vi "Get_DeviceInformation.vi"(8 "error in (no error)":errorcluster, 11 "Avantes in":refnum<class "Avantes.lvclass">) -> (0 "error out":errorcluster, 2 "Array":string[](array[string]), 3 "Avantes out":refnum<class "Avantes.lvclass">)   [LabVIEW 2020, in "Avantes.lvclass"]
uses:
  <instrlib>/Classes/CCD/Avantes/Avantes.lvclass
panel:
  in  "Enum":enum16{"Intern", "Extern"}(ring)
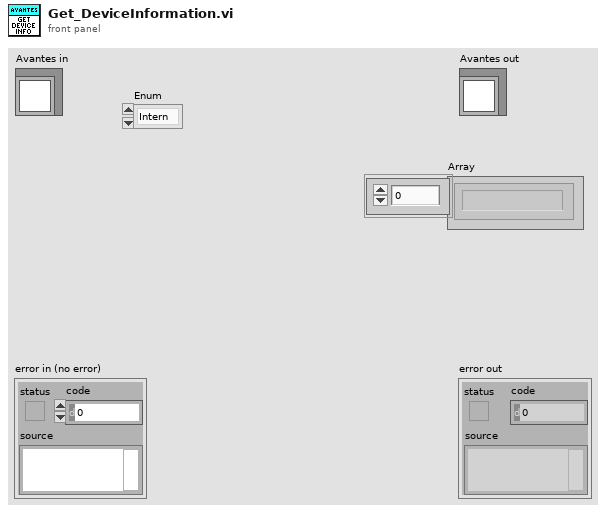
[diagram p1: front panel]
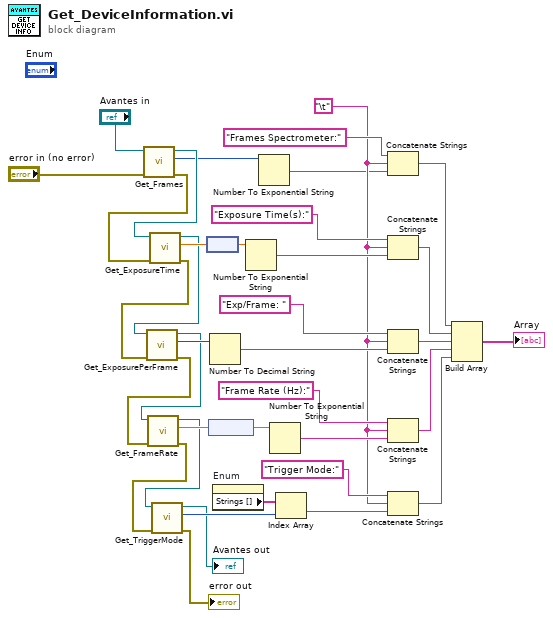
[diagram p0: block diagram]
diagram:
  w3 = "\t"
  n1 = call-dynamic "Get_Frames.vi"("error in (no error)"="error in (no error)", "Avantes in"="Avantes in") -> ("error out"=w6:errorcluster, "Frames"=w5:i32, "Avantes out"=w9:refnum<class "Avantes.lvclass">)  [unwired: 7 in]
  n2 = call-dynamic "Get_ExposureTime.vi"("error in (no error)"=w6, "Avantes in"=w9) -> ("error out"=w31:errorcluster, "Exposure Time"=w37:dbl[unit], "Avantes out"=w32:refnum<class "Avantes.lvclass">)  [unwired: 7 in]
  n3 = call-dynamic "Get_ExposurePerFrame.vi"("error in (no error)"=w31, "Avantes in"=w32) -> ("error out"=w27:errorcluster, "Exposure per Frame"=w33:i32, "Avantes out"=w28:refnum<class "Avantes.lvclass">)  [unwired: 7 in]
  n4 = call-dynamic "Get_FrameRate.vi"("error in (no error)"=w27, "Avantes in"=w28) -> ("error out"=w21:errorcluster, "Frame Rate"=w26:dbl[unit], "Avantes out"=w22:refnum<class "Avantes.lvclass">)  [unwired: 7 in]
  n5 = call-dynamic "Get_TriggerMode.vi"("error in (no error)"=w21, "Avantes in"=w22) -> ("error out"=→"error out":errorcluster, "Trigger Mode"=w19:u16, "Avantes out"=→"Avantes out":refnum<class "Avantes.lvclass">)  [unwired: 7 in]
  n6 = node(w37) -> (w36:dbl)
  n7 = node(w26) -> (w25:dbl)
  n8 = Number To Decimal String(number=w33) -> (decimal integer string=w29:string)  [unwired: 1 in]
  n9 = property on="Enum" class="Enum (strict)"() -> ("Strings []"=w20:string[])  [unwired: 2 in, 2 out]
  n10 = Number To Exponential String(number=w36) -> (E-format string=w35:string)  [unwired: 3 in]
  n11 = Number To Exponential String(number=w5) -> (E-format string=w2:string)  [unwired: 3 in]
  n12 = Number To Exponential String(number=w25) -> (E-format string=w24:string)  [unwired: 3 in]
  n13 = Index Array(array=w20, index=w19) -> (element=w18:string)
  n14 = Concatenate Strings("Frames Spectrometer:", w3, w2) -> (w1:string)
  n15 = Concatenate Strings("Exposure Time(s):", w3, w35) -> (w14:string)
  n16 = Concatenate Strings("Exp/Frame: ", w3, w29) -> (w13:string)
  n17 = Concatenate Strings("Frame Rate (Hz):", w3, w24) -> (w12:string)
  n18 = Concatenate Strings("Trigger Mode:", w3, w18) -> (w11:string)
  n19 = Build Array(w1, w14, w13, w12, w11) -> (→"Array":string[])
